vi "ConfigureControllerGain.vi"(0 "axis in":cluster{"keyHandle":u32, "nodeId":u16}={"keyHandle"=0, "nodeId"=1}, 11 "error in (no error)":errorcluster) -> (4 "axis out":cluster{"keyHandle":u32, "nodeId":u16}={"keyHandle"=0, "nodeId"=1}, 15 "error out":errorcluster)   [LabVIEW 2017, in "maxonEPOS.lvlib"]
doc: "<B>ConfigureVelocityRegulator</B> writes the velocity regulation gain parameters to the device."
uses:
  Examples/maxonEPOS.lvlib
panel:
  in  "value":u64
  in  "controller gain":cluster{"controller":u16, "gain":u16}={"controller"=21, "gain"=2} {"controller" items=[""=0, "PI Current Controller"=1, "PI Velocity Controller"=10, "PI Velocity Controller with Observer"=11, "PID Position Controller"=20, "Dual Loop Position Controller"=21]; "gain" items=[""=0, "P-Gain"=1, "I-Gain"=2, "D-Gain"=3, "Feedforward Velocity Gain"=10, "Feedforward Acceleration Gain"=11, "Theta Gain"=20, "Omega Gain"=21, "Tau Gain"=22, "P Gain low"=101, "P Gain high"=102, "Gain Scheduling Weight"=110, "Filter Coefficient A"=120, "Filter Coefficient B"=121, "Filter Coefficient C"=122, "Filter Coefficient D"=123, "Filter Coefficient E"=124]}
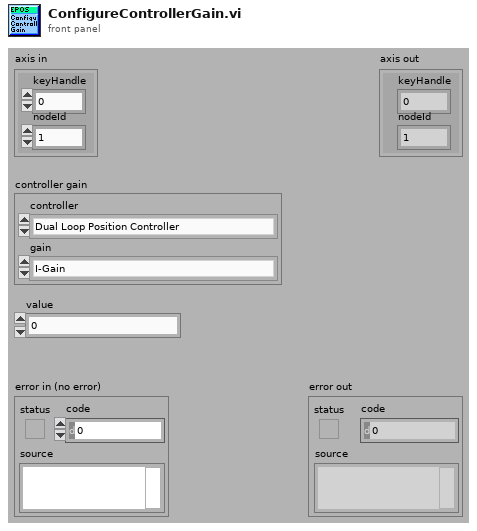
[diagram p1: front panel]
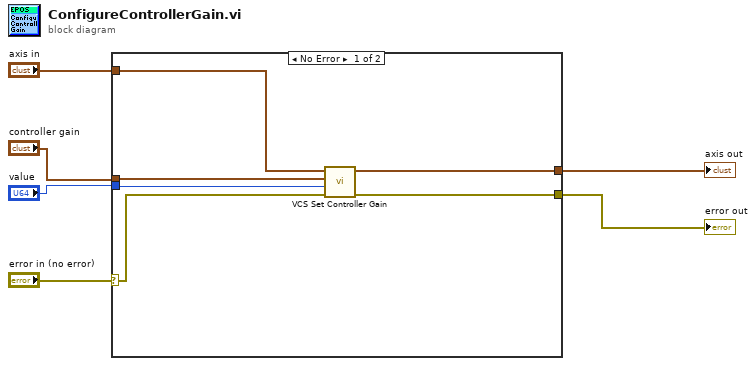
[diagram p0: block diagram]
diagram:
  n1 = case shown="No Error" "error in (no error)" {
    selector: "error in (no error)" -> [w10 w14]
    tunnel: [w12 w14] -> w5
    tunnel: [w11 w13] -> w4
    tunnel: "axis in" -> [w9 w13]
    tunnel: "controller gain" -> [w8 _]
    tunnel: "value" -> [w7 _]
    frame No Error {
      n2 = call "VCS Set Controller Gain.vi"("error in (no error)"=w10, "value"=w7, "controller gain"=w8, "axis in"=w9) -> ("error out"=w12:errorcluster, "axis out"=w11:cluster{"keyHandle":u32, "nodeId":u16})  [unwired: 6 in]
    }
    frame Error {
    }
  }
  "error out" <- w5
  "axis out" <- w4
